vi "Async.Processes.Report.vi"(8 "error in":errorcluster, 10 "Stop Async on Error?":bool, 11 "Process in":refnum<class "Process.lvclass">) -> (2 "Stop":bool, 3 "Process out":refnum<class "Process.lvclass">)   [LabVIEW 2027, in "VS Inline Async API (Express).lvlib" / "Process.lvclass"]
uses:
  Process.lvclass
  Process.lvclass/Process.ctl
  VS Inline Async API (Express).lvlib
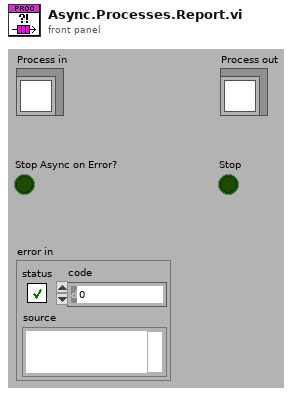
[diagram p1: front panel]
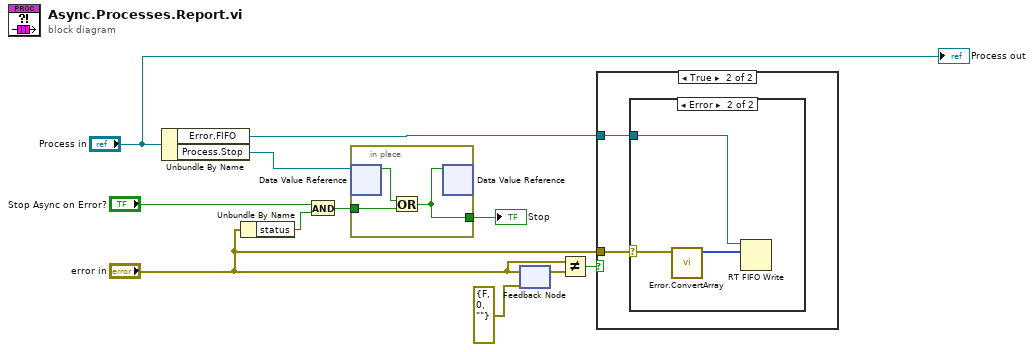
[diagram p0: block diagram]
diagram:
  n1 = Unbundle By Name("Process in") -> ("Error.FIFO"=w9:refnum<k33>, "Process.Stop"=w3:refnum<data-value>)
  n2 = Unbundle By Name("error in") -> ("status"=w7:bool)
  n3 = And(x="Stop Async on Error?", y=w7) -> (x .and. y?=w6:bool)
  n4 = in-place {
    in-place-border: [w12] -> w5
    in-place-border: w6 -> [w13]
    n5 = in-place-dvr #1(w3) -> (w14:bool)  [unwired: 1 out]
    n6 = Or(x=w14, y=w13) -> (x .or. y?=w12:bool)
    n7 = in-place-dvr #1(w12) -> ()  [unwired: 2 out]
  }
  "Stop" <- w5
  n8 = feedback #2(errorcluster {"status"=FALSE, "code"=0, "source"=""} ("Error")) -> (w10:errorcluster)
  n9 = feedback-in #2("error in") -> ()
  n10 = Not Equal?(x="error in", y=w10) -> (x != y?=w11:bool)
  n11 = case shown="True" w11 {
    tunnel: w9 -> [_ w16]
    tunnel: "error in" -> [_ w15]
    frame False {
    }
    frame True {
      n12 = case shown="Error" w15 {
        selector: w15 -> [_ w18]
        tunnel: w16 -> [_ w19]
        frame No Error {
        }
        frame Error {
          n13 = call "Error.ConvertArray.vi"("error in"=w18) -> ("Msg"=w17:u8[])  [unwired: 10 in]
          n14 = RT FIFO Write(0:w19, 1:w17) -> ()  [unwired: 3 in, 4 out]
        }
      }
    }
  }
  "Process out" <- "Process in"
